vi "MainNR.vi"(10 "JQMHStartup":refnum<class "RQMHStartup.lvclass">, 11 "NewTemplate in":refnum<class "UIManager.lvclass">) -> ()   [LabVIEW 2024, in "UIManager.lvclass"]
uses:
  UIManager.lvclass
  C:/Github/JQMH/JQMHCore/Module/RQMHModule.lvclass
  JQMHCore/JQMHStartup/RQMHStartup.lvclass
  Shell/Shell.lvclass
  Layout/Layout.lvclass
  JQMHCore/Module/RQMHModule.lvclass
  Message Queue_class/RQMHMessageQueue.lvclass/RQMHMessageQueue.ctl
  JQMHCore/Module/InitialiseReplyArgs.ctl
  <vilib>/Utility/miscctls.llb/LVPointTypeDef.ctl
  JQMHCore/Module/RQMHModule.lvclass/RQMHModule.ctl
  Do Something ReplyArgs.ctl
  Do Something Args.ctl
  Prepare Args.ctl
  Prepare ReplyArgs.ctl
  Show ReplyArgs.ctl
  Show Args.ctl
  Add Eng Panel Args.ctl
  Add Eng Panel ReplyArgs.ctl
  Message Queue_class/Delacor_lib_QMH_Enqueue Message (Single).vi
  JQMHCore/Module/Read ModuleName.vi
  JQMHCore/Module/Read External Start.vi
  TitleBar/TitleBar.lvclass
  Header/Header.lvclass
  JQMHCore/Module/Show In Subpanel.vi
  JQMHCore/Module/Show Front Panel.vi
  Message Queue_class/RQMHMessageQueue.lvclass
  JQMHCore/Shared/RQMHShared.lvlib
  C:/Github/JQMH/ModuleTemplates/TitleBar/TitleBar.lvclass
  C:/Github/JQMH/ModuleTemplates/Header/Header.lvclass
  C:/Github/JQMH/ModuleTemplates/Shell/Shell.lvclass
  C:/Github/JQMH/ModuleTemplates/Layout/Layout.lvclass
panel:
  out "error out":errorcluster
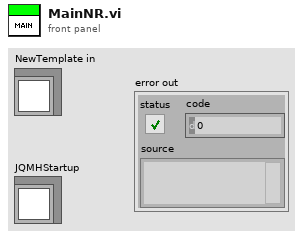
[diagram p1: front panel]
types:
  T1 = typedef "RQMHModule.lvclass/StandardBroadcasts.ctl" = cluster{"Died":refnum<user-event>, "Started":refnum<user-event>}
  T2 = typedef "Header.lvclass/Broadcast Events--cluster.ctl" = cluster{"Stopped":refnum<user-event>, "Menu Item Selected":refnum<user-event>}
  T3 = typedef "TitleBar.lvclass/Broadcast Events--cluster.ctl" = cluster{"Stopped":refnum<user-event>, "Maximise":refnum<user-event>, "Minimise":refnum<user-event>, "ClosePress":refnum<user-event>}
  T4 = typedef "UIManager.lvclass/Request Events--cluster.ctl" = cluster{"Do Something":refnum<user-event>, "Prepare":refnum<user-event>, "Show":refnum<user-event>, "AddEngPanel":refnum<user-event>, "Add Eng Panel":refnum<user-event>}
  T5 = cluster{"Stop Module":refnum<user-event>, "Requests":T4}
  T6 = cluster{"Shell":refnum<class "Shell.lvclass">, "Layout":refnum<class "Layout.lvclass">, "TitleBar":refnum<class "TitleBar.lvclass">, "Header":refnum<class "Header.lvclass">, "EngPanels":map{string, refnum<class "RQMHModule.lvclass">}}
  T7 = typedef "LVPointTypeDef.ctl" = cluster{"Horizontal":i16, "Vertical":i16}
  T8 = enum32{"Invalid", "Standard", "Closed", "Hidden", "Minimized", "Maximized"}
  T9 = typedef "RQMHModule.lvclass/InitialiseReplyArgs.ctl" = cluster{"Did Init?":bool}
  T10 = typedef "UIManager.lvclass/Do Something Args.ctl" = cluster{"Msg":string}
  T11 = typedef "UIManager.lvclass/Do Something ReplyArgs.ctl" = cluster{"Value":dbl, "Boolean":bool}
  T12 = typedef "UIManager.lvclass/Prepare ReplyArgs.ctl" = cluster{"null":bool}
  T13 = typedef "UIManager.lvclass/Prepare Args.ctl" = cluster{"String":string}
  T14 = typedef "UIManager.lvclass/Show Args.ctl" = cluster{"String":string}
  T15 = typedef "UIManager.lvclass/Show ReplyArgs.ctl" = cluster{"Boolean":bool}
  T16 = typedef "UIManager.lvclass/Add Eng Panel ReplyArgs.ctl" = cluster{"null":bool}
  T17 = typedef "UIManager.lvclass/Add Eng Panel Args.ctl" = cluster{"EngPanel":refnum<class "RQMHModule.lvclass">, "Name":string}
  T18 = typedef "RQMHModule.lvclass/Reply.ctl" = cluster{"Expects Reply":bool, "Reply":refnum<notifier>}
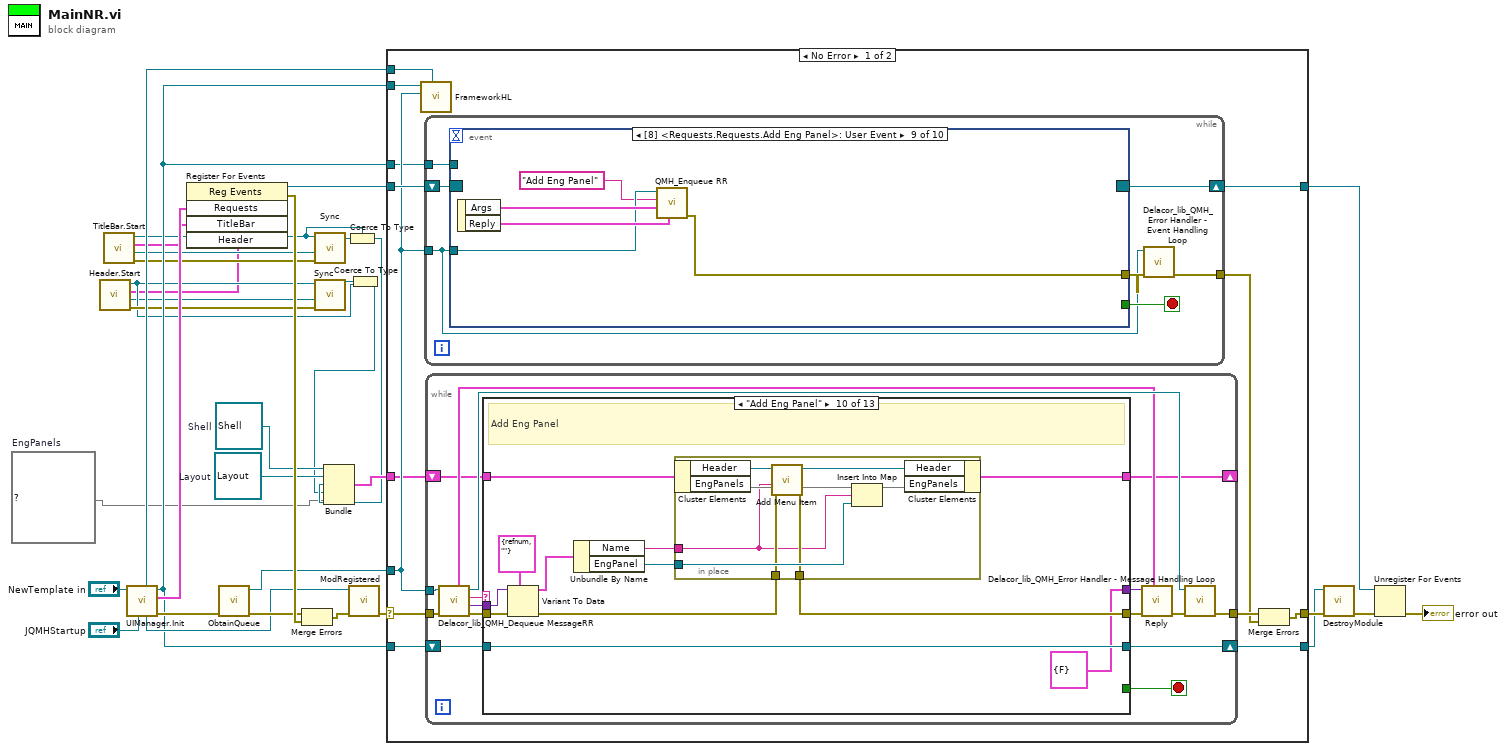
[diagram p0: block diagram]
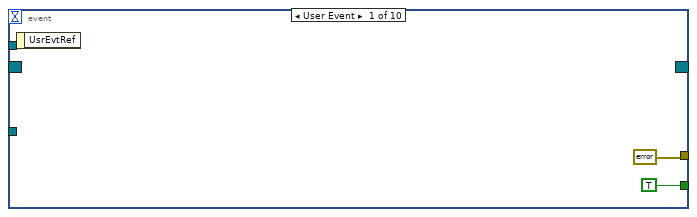
[diagram p2: hidden frame]
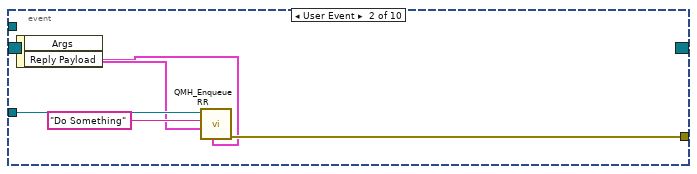
[diagram p3: hidden frame]
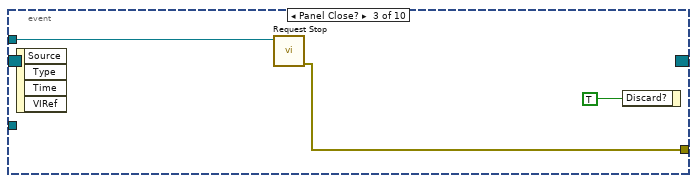
[diagram p4: hidden frame]
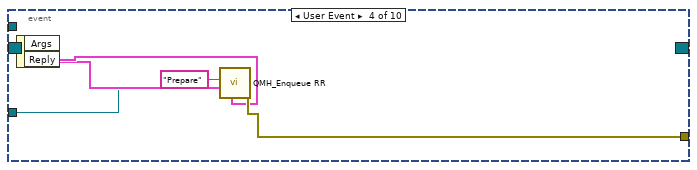
[diagram p5: hidden frame]
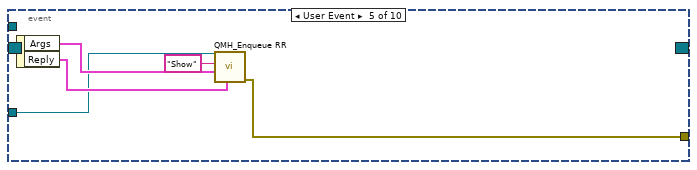
[diagram p6: hidden frame]
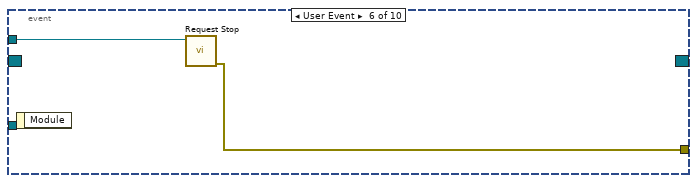
[diagram p7: hidden frame]
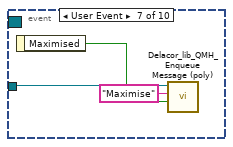
[diagram p8: hidden frame]
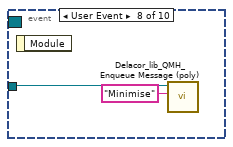
[diagram p9: hidden frame]
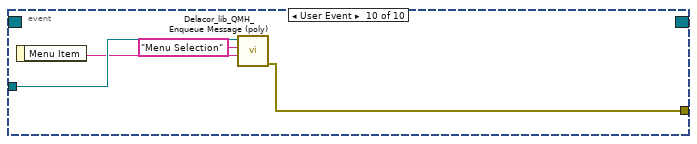
[diagram p10: hidden frame]
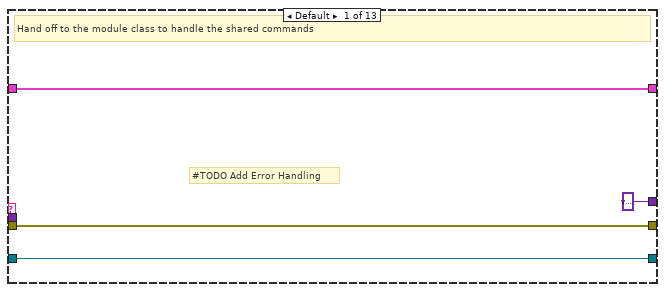
[diagram p11: hidden frame]
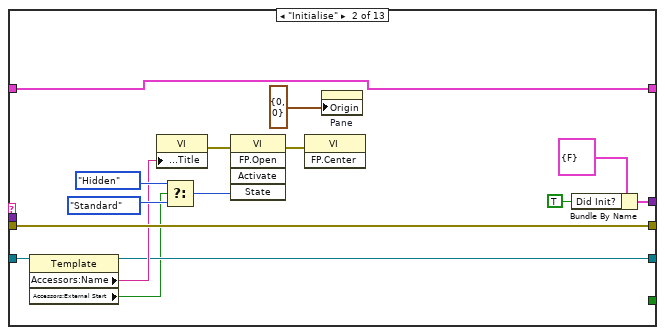
[diagram p12: hidden frame]
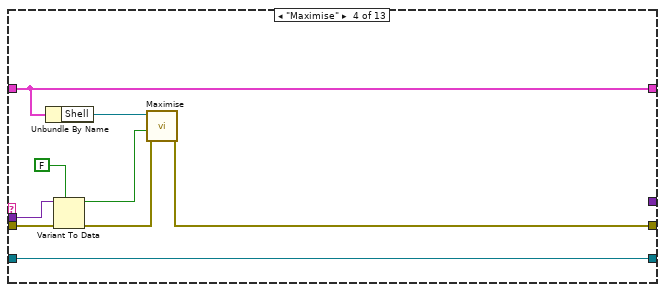
[diagram p14: hidden frame]
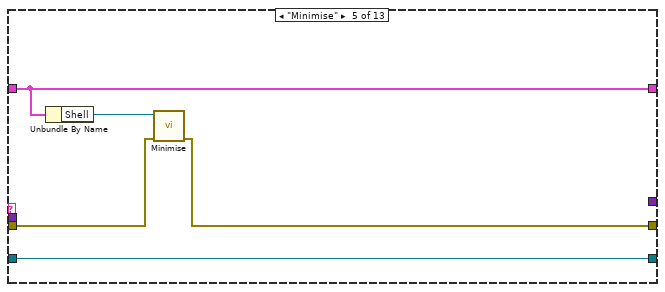
[diagram p15: hidden frame]
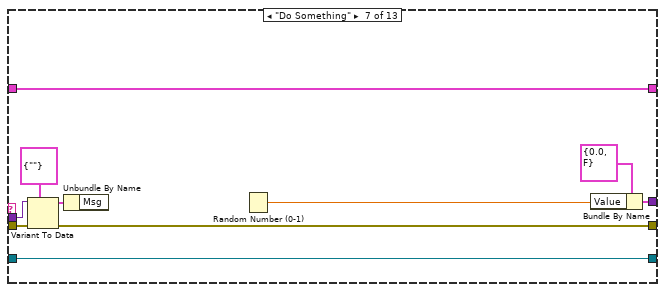
[diagram p17: hidden frame]
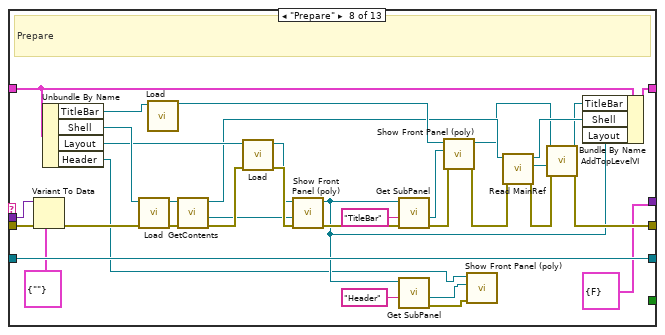
[diagram p18: hidden frame]
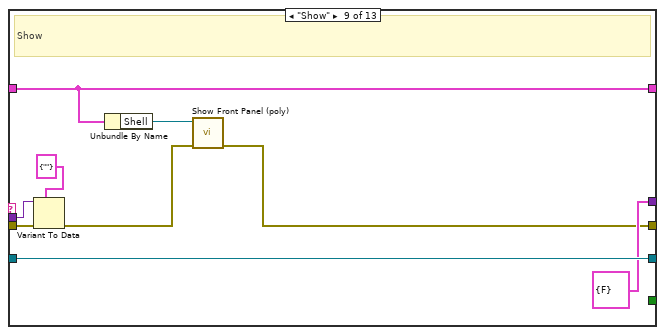
[diagram p19: hidden frame]
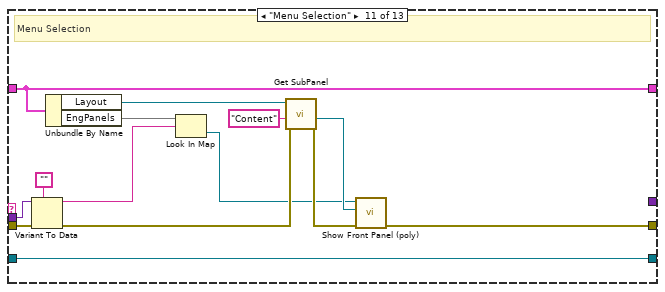
[diagram p20: hidden frame]
diagram:
  w2 = map{string, refnum<class "RQMHModule.lvclass">} {}  # EngPanels
  w14 = refnum<class "Layout.lvclass"> refnum  # Layout
  w16 = refnum<class "Shell.lvclass"> refnum  # Shell
  n1 = call "Header.Start.vi"() -> ("error out"=w5:errorcluster, "StartupHandshake out"=w3:refnum<class "RQMHStartup.lvclass">, 2:"Header"=w1:cluster{"Broadcasts":T1, "Broadcasts":T2}, 3:"Header"=w4:refnum<class "Header.lvclass">)  [unwired: 8 in]
  n2 = call "TitleBar.Start.vi"() -> ("error out"=w11:errorcluster, "StartupHandshake out"=w12:refnum<class "RQMHStartup.lvclass">, 2:"TitleBar"=w13:cluster{"Broadcasts":T1, "Broadcasts":T3}, 3:"TitleBar"=w8:refnum<class "TitleBar.lvclass">)  [unwired: 8 in]
  n3 = call "UIManager.Init.vi"("JQMHStartup in"="JQMHStartup", "NewTemplate in"="NewTemplate in") -> ("error out"=w27:errorcluster, "Requests"=w18:T5, "NewTemplate out"=w17:refnum<class "UIManager.lvclass">, "JQMHStartup out"=w25:refnum<class "RQMHStartup.lvclass">, "StandardRequests"=w21:refnum<event-registration>)  [unwired: 4 in, 1 out]
  n4 = register-events(w18, w13, w1) -> (reference out=w20:refnum<event-registration>, error out=w34:errorcluster)  [unwired: 2 in]
  n5 = call "ObtainQueue.vi"("error in"=w27) -> ("error out"=w26:errorcluster, "Message Queue"=w22:refnum<class "RQMHMessageQueue.lvclass">)  [unwired: 9 in]
  n6 = Merge Errors(w26, w34) -> (w23:errorcluster)
  n7 = call "Sync.vi"("error in (no error)"=w11, "StartupHandshake out"=w12, "JQMHCore in"=w8) -> ("JQMHCore out"=w9:refnum<class "TitleBar.lvclass">)  [unwired: 7 in, 1 out]
  n8 = call "Sync.vi"("error in (no error)"=w5, "StartupHandshake out"=w3, "JQMHCore in"=w4) -> ("JQMHCore out"=w6:refnum<class "Header.lvclass">)  [unwired: 7 in, 1 out]
  n9 = Coerce To Type(0:w9, 1:w8) -> (2:w10:refnum<class "TitleBar.lvclass">)
  n10 = call "ModRegistered.vi"("error in (no error)"=w23, "JQMHStartup in"=w25) -> ("error out"=w24:errorcluster)  [unwired: 9 in]
  n11 = Coerce To Type(0:w6, 1:w4) -> (2:w7:refnum<class "Header.lvclass">)
  n12 = Bundle("Shell"=w16, "Layout"=w14, "TitleBar"=w10, "Header"=w7, "EngPanels"=w2) -> (w15:T6)  [unwired: 1 in]
  n13 = case "RQMH_MAIN" shown="No Error" w24 {
    selector: w24 -> [w44 w257]
    tunnel: w17 -> [w47 w256]
    tunnel: [w46 w259] -> w33
    tunnel: w20 -> [w45 w259]
    tunnel: w22 -> [w38 w258]
    tunnel: [w43 w256] -> w19
    tunnel: [w40 w255] -> w30
    tunnel: w17 -> [w39 _]
    tunnel: w21 -> [w37 w254]
    tunnel: w17 -> [w36 _]
    tunnel: w15 -> [w35 _]
    frame No Error {
      n14 = call-dynamic "FrameworkHL.vi"("StandardRequests"=w37, "Message Queue"=w38, "JQMHModule in"=w39) -> ()  [unwired: 9 in]
      n15 = while {
        shift-right: [w54] -> w46
        shift-left: w45 -> [w49]
        tunnel: w38 -> [w50]
        tunnel: [w51] -> w41
        tunnel: w36 -> [w48]
        stop <- w53 stop-if-true
        n16 = event "RQMH_EVENT_MAIN" shown="[8] <Requests.Requests.Add Eng Panel>: User Event" {
          selector: w49 -> [_ _ _ _ _ _ _ _ _ _]
          dyn-events: [_ _ _ _ _ _ _ _ _ _] -> w54
          timeout: _ -> [_ _ _ _ _ _ _ _ _ _]
          tunnel: [TRUE _ _ _ _ _ _ _ _ _] -> w53
          tunnel: w50 -> [_ w61 _ w66 w71 _ w79 w81 w83 w90]
          tunnel: [errorcluster {"status"=FALSE, "code"=0, "source"=""} ("error out") w58 w62 w69 w74 w75 _ _ w86 w87] -> w52
          tunnel: w48 -> [_ _ w63 _ _ w76 _ _ _ _]
          event User Event {
            n17 = event-data() -> ()  [unwired: 1 in, 1 out]
          }
          event User Event {
            n18 = event-data() -> ("Args"=w59:T10, "Reply Payload"=w57:T18)  [unwired: 1 in]
            n19 = call "QMH_Enqueue RR.vi"("Reply"=w57, "Message Data"=w59, "Message"="Do Something", "Message Queue in"=w61) -> ("error out"=w58:errorcluster)  [unwired: 6 in, 1 out]
          }
          event Panel Close? {
            n20 = event-data() -> ()  [unwired: 1 in, 4 out]
            n21 = call "Request Stop.vi"("module in"=w63) -> ("error out"=w62:errorcluster)  [unwired: 9 in, 1 out]
            n22 = event-data("Discard?"=TRUE) -> ()  [unwired: 1 in, 1 out]
          }
          event User Event {
            n23 = event-data() -> ("Args"=w67:T13, "Reply"=w68:T18)  [unwired: 1 in]
            n24 = call "QMH_Enqueue RR.vi"("Reply"=w68, "Message Data"=w67, "Message"="Prepare", "Message Queue in"=w66) -> ("error out"=w69:errorcluster)  [unwired: 6 in, 1 out]
          }
          event User Event {
            n25 = event-data() -> ("Args"=w72:T14, "Reply"=w73:T18)  [unwired: 1 in]
            n26 = call "QMH_Enqueue RR.vi"("Reply"=w73, "Message Data"=w72, "Message"="Show", "Message Queue in"=w71) -> ("error out"=w74:errorcluster)  [unwired: 6 in, 1 out]
          }
          event User Event {
            n27 = event-data() -> ()  [unwired: 1 in, 1 out]
            n28 = call "Request Stop.vi"("module in"=w76) -> ("error out"=w75:errorcluster)  [unwired: 9 in, 1 out]
          }
          event User Event {
            n29 = event-data() -> ("Maximised"=w77:bool)  [unwired: 1 in]
            n30 = call-poly "Delacor_lib_QMH_Enqueue Message (poly).vi"("Message Data"=w77, "Message"="Maximise", "Message Queue in"=w79) -> ()  [unwired: 7 in, 2 out]
          }
          event User Event {
            n31 = event-data() -> ()  [unwired: 1 in, 1 out]
            n32 = call-poly "Delacor_lib_QMH_Enqueue Message (poly).vi"("Message"="Minimise", "Message Queue in"=w81) -> ()  [unwired: 8 in, 2 out]
          }
          event User Event {
            n33 = event-data() -> ("Args"=w84:T17, "Reply"=w85:T18)  [unwired: 1 in]
            n34 = call "QMH_Enqueue RR.vi"("Reply"=w85, "Message Data"=w84, "Message"="Add Eng Panel", "Message Queue in"=w83) -> ("error out"=w86:errorcluster)  [unwired: 6 in, 1 out]
          }
          event User Event {
            n35 = event-data() -> ("Menu Item"=w89:string)  [unwired: 1 in]
            n36 = call-poly "Delacor_lib_QMH_Enqueue Message (poly).vi"("Message Data"=w89, "Message"="Menu Selection", "Message Queue in"=w90) -> ("error out"=w87:errorcluster)  [unwired: 7 in, 1 out]
          }
        }
        n37 = call-dynamic "Delacor_lib_QMH_Error Handler - Event Handling Loop.vi"("error in"=w52, "Message Queue in"=w50) -> ("dup error in"=w51:errorcluster)  [unwired: 8 in, 1 out]
      }
      n38 = while {
        tunnel: w38 -> [w101]
        tunnel: w44 -> [w100]
        shift-right: [w103] -> w43
        shift-left: w47 -> [w104]
        tunnel: [w102] -> w42
        shift-right: [w91] -> _
        shift-left: w35 -> [w92]
        stop <- w106 stop-if-true
        n39 = call-dynamic "Delacor_lib_QMH_Dequeue MessageRR.vi"("error in"=w100, "Message Queue in"=w101) -> ("error out"=w99:errorcluster, "Message Data"=w97:variant, "Message"=w98:string, "Message Queue out"=w105:refnum<class "RQMHMessageQueue.lvclass">, "Reply"=w93:T18)  [unwired: 5 in]
        n40 = case "RQMH_MESSAGE_CASES" shown="\"Add Eng Panel\"" w98 {
          tunnel: [_ _ _ _ _ _ _ _ _ _ _ _ TRUE] -> w106
          tunnel: w104 -> [w109 w113 w127 w136 w142 w144 w155 w189 w198 w210 w232 w238 w252]
          tunnel: w97 -> [_ _ _ w134 _ _ w151 w188 w197 w209 w231 w236 _]
          tunnel: w99 -> [w110 w125 w128 w137 w138 w145 w150 w190 w199 w211 w233 w240 w251]
          tunnel: [w110 w125 w128 w130 w139 w145 w149 w164 w191 w201 w221 w239 w251] -> w96
          tunnel: [w109 w114 w127 w136 w142 w144 w155 w189 w198 w210 w232 w237 w252] -> w103
          tunnel: [variant w124 _ _ _ _ w154 T12 {"null"=FALSE} ("Prepare ReplyArgs") T15 {"Boolean"=FALSE} ("RQMH_MHL_REPLY_PL") T16 {"null"=FALSE} _ w235 _] -> w94
          tunnel: w92 -> [w107 w111 w126 w135 w141 w143 w146 w184 w194 w208 w229 w234 w250]
          tunnel: [w107 w111 w126 w135 w141 w143 w146 w185 w194 w205 w229 w234 w250] -> w91
          frame Default {
            # "#TODO Add Error Handling"
            # "Hand off to the module class to handle the shared commands"
          }
          frame "Initialise" {
            n41 = property class="Template"(reference=w113) -> (reference out=w114:refnum<class "UIManager.lvclass">, "Accessors:Name"=w115:string, "Accessors:External Start"=w112:bool)  [unwired: 1 in, 1 out]
            n42 = property on="Property Node" class="VI"("Front Panel.Title"=w115) -> (error out=w122:errorcluster)  [unwired: 2 in, 1 out]
            n43 = Select(t=T8."Hidden" ("State"), s=w112, f=T8."Standard" ("State")) -> (s? t:f=w118:T8)
            n44 = invoke on="Invoke Node" class="VI" method="FP.Open"(error in=w122, "State"=w118) -> (error out=w121:errorcluster)  [unwired: 3 in, 4 out]
            n45 = invoke on="Invoke Node" class="VI" method="FP.Center"(error in=w121) -> ()  [unwired: 2 in, 3 out]
            n46 = property on="Pane" class="Pane"("Origin"=T7 {"Horizontal"=0, "Vertical"=0}) -> ()  [unwired: 2 in, 2 out]
            n47 = Bundle By Name(cluster=T9 {"Did Init?"=FALSE} ("Args"), "Did Init?"=TRUE) -> (w124:T9)
          }
          frame "---Internal---" {
          }
          frame "Maximise" {
            n48 = Unbundle By Name(w135) -> ("Shell"=w132:refnum<class "Shell.lvclass">)
            n49 = Variant To Data(error in=w137, type=FALSE, Variant=w134) -> (data=w129:bool, error out=w131:errorcluster)
            n50 = call "Maximise.vi"("error in (no error)"=w131, "Maximise"=w129, "module in"=w132) -> ("error out"=w130:errorcluster)  [unwired: 6 in, 2 out]
          }
          frame "Minimise" {
            n51 = Unbundle By Name(w141) -> ("Shell"=w140:refnum<class "Shell.lvclass">)
            n52 = call "Minimise.vi"("error in (no error)"=w138, "module in"=w140) -> ("error out"=w139:errorcluster)  [unwired: 7 in, 2 out]
          }
          frame "---Module Specific---" {
          }
          frame "Do Something" {
            n53 = Variant To Data(error in=w150, type=T10 {"Msg"=""} ("Do Something Args"), Variant=w151) -> (data=w147:T10, error out=w149:errorcluster)
            n54 = Unbundle By Name(w147) -> ()  [unwired: 1 out]
            n55 = Random Number (0-1)() -> (number: 0 to 1=w152:dbl)
            n56 = Bundle By Name(cluster=T11 {"Value"=0.0, "Boolean"=FALSE}, "Value"=w152) -> (w154:T11)
          }
          frame "Prepare" {
            # "Prepare"
            n57 = Variant To Data(error in=w190, type=T13 {"String"=""} ("RQMH_MHL_MSG_PL"), Variant=w188) -> (error out=w186:errorcluster)  [unwired: 1 out]
            n58 = Unbundle By Name(w184) -> ("TitleBar"=w175:refnum<class "TitleBar.lvclass">, "Shell"=w183:refnum<class "Shell.lvclass">, "Layout"=w182:refnum<class "Layout.lvclass">, "Header"=w158:refnum<class "Header.lvclass">)
            n59 = call "Load.vi"("error in (no error)"=w186, "RQMHModule in"=w183) -> ("error out"=w180:errorcluster, "RQMHModule out"=w181:refnum<class "Shell.lvclass">)  [unwired: 8 in]
            n60 = call "Load.vi"("RQMHModule in"=w175) -> ("RQMHModule out"=w172:refnum<class "TitleBar.lvclass">)  [unwired: 9 in, 1 out]
            n61 = call "GetContents.vi"("error in (no error)"=w180, "module in"=w181) -> ("error out"=w179:errorcluster, "Sub Panel"=w177:refnum<vi>, "module out"=w168:refnum<class "Shell.lvclass">)  [unwired: 6 in, 1 out]
            n62 = call "Load.vi"("error in (no error)"=w179, "RQMHModule in"=w182) -> ("error out"=w178:errorcluster, "RQMHModule out"=w176:refnum<class "Layout.lvclass">)  [unwired: 8 in]
            n63 = call-poly "Show Front Panel (poly).vi"("error in (no error)"=w178, "Sub Panel"=w177, "JQMHCore in"=w176) -> ("error out"=w174:errorcluster, "JQMHCore out"=w159:refnum<class "Layout.lvclass">)  [unwired: 7 in]
            n64 = call "Get SubPanel.vi"("error in (no error)"=w174, "Panel Name"="TitleBar", "module in"=w159) -> ("error out"=w170:errorcluster, "Sub Panel"=w171:refnum<vi>)  [unwired: 5 in, 2 out]
            n65 = call "Get SubPanel.vi"("Panel Name"="Header", "module in"=w159) -> ("error out"=w156:errorcluster, "Sub Panel"=w157:refnum<vi>)  [unwired: 6 in, 2 out]
            n66 = call-poly "Show Front Panel (poly).vi"("error in (no error)"=w170, "Sub Panel"=w171, "JQMHCore in"=w172) -> ("error out"=w163:errorcluster, "JQMHCore out"=w166:refnum<class "TitleBar.lvclass">)  [unwired: 7 in]
            n67 = call-poly "Show Front Panel (poly).vi"("error in (no error)"=w156, "Sub Panel"=w157, "JQMHCore in"=w158) -> ()  [unwired: 7 in, 2 out]
            n68 = call "Read MainRef.vi"("error in (no error)"=w163, "RQMHModule in"=w168) -> ("error out"=w162:errorcluster, "MainRef"=w169:refnum<vi>, "RQMHModule out"=w167:refnum<class "Shell.lvclass">)  [unwired: 7 in]
            n69 = call "AddTopLevelVI.vi"("error in (no error)"=w162, "MainRef"=w169, "module in"=w166) -> ("error out"=w164:errorcluster, "module out"=w165:refnum<class "TitleBar.lvclass">)  [unwired: 6 in, 1 out]
            n70 = Bundle By Name(cluster=w184, "TitleBar"=w165, "Shell"=w167, "Layout"=w159) -> (w185:T6)
          }
          frame "Show" {
            # "Show"
            n71 = Variant To Data(error in=w199, type=T14 {"String"=""} ("RQMH_MHL_MSG_PL"), Variant=w197) -> (error out=w192:errorcluster)  [unwired: 1 out]
            n72 = Unbundle By Name(w194) -> ("Shell"=w193:refnum<class "Shell.lvclass">)
            n73 = call-poly "Show Front Panel (poly).vi"("error in (no error)"=w192, "JQMHCore in"=w193) -> ("error out"=w191:errorcluster)  [unwired: 8 in, 1 out]
          }
          frame "Add Eng Panel" {
            # "Add Eng Panel"
            n74 = Variant To Data(error in=w211, type=T17 {"EngPanel"=refnum, "Name"=""} ("RQMH_MHL_MSG_PL"), Variant=w209) -> (data=w206:T17, error out=w202:errorcluster)
            n75 = Unbundle By Name(w206) -> ("Name"=w204:string, "EngPanel"=w203:refnum<class "RQMHModule.lvclass">)
            n76 = in-place {
              in-place-border: w204 -> [w212]
              in-place-border: w203 -> [w217]
              in-place-border: w202 -> [w214]
              in-place-border: [w213] -> w201
              n77 = in-place-cluster #1(w208) -> ("Header"=w216:refnum<class "Header.lvclass">, "EngPanels"=w219:map{string, refnum<class "RQMHModule.lvclass">})
              n78 = call "Add Menu Item.vi"("error in (no error)"=w214, "Item"=w212, "module in"=w216) -> ("error out"=w213:errorcluster, "module out"=w215:refnum<class "Header.lvclass">)  [unwired: 7 in]
              n79 = Insert Into Map(map in=w219, key=w212, value=w217) -> (map out=w218:map{string, refnum<class "RQMHModule.lvclass">})  [unwired: 2 out]
              n80 = in-place-cluster #1("Header"=w215, "EngPanels"=w218) -> (w205:T6)
            }
          }
          frame "Menu Selection" {
            # "Menu Selection"
            n81 = Variant To Data(error in=w233, type="", Variant=w231) -> (data=w227:string, error out=w223:errorcluster)
            n82 = Unbundle By Name(w229) -> ("Layout"=w224:refnum<class "Layout.lvclass">, "EngPanels"=w228:map{string, refnum<class "RQMHModule.lvclass">})
            n83 = Look In Map(map=w228, key=w227) -> (value=w220:refnum<class "RQMHModule.lvclass">)  [unwired: 1 in, 1 out]
            n84 = call "Get SubPanel.vi"("error in (no error)"=w223, "Panel Name"="Content", "module in"=w224) -> ("error out"=w222:errorcluster, "Sub Panel"=w226:refnum<vi>)  [unwired: 5 in, 2 out]
            n85 = call-poly "Show Front Panel (poly).vi"("error in (no error)"=w222, "Sub Panel"=w226, "JQMHCore in"=w220) -> ("error out"=w221:errorcluster)  [unwired: 7 in, 1 out]
          }
          frame "---Copy This Frame---" {
            # "This is the frame that is copied when scripting\nDO NOT CHANGE NAME OF FRAME"
            n86 = disable-structure shown="Disabled" {
              disable-tunnel: w240 -> [w244 w249]
              disable-tunnel: [w245 w249] -> w239
              disable-tunnel: w238 -> [w247 w248]
              disable-tunnel: [w247 w248] -> w237
              disable-tunnel: w236 -> [w246 _]
              disable-tunnel: [w242 _] -> w235
              frame Disabled {
                # "Anything in this diagram will be used when adding a new request"
                n87 = Variant To Data(error in=w244, type=cluster{string} {""} ("RQMH_MHL_MSG_PL"), Variant=w246) -> (error out=w245:errorcluster)  [unwired: 1 out]
                n88 = Bundle By Name(cluster=cluster{string} {""} ("RQMH_MHL_REPLY_PL")) -> (w242:cluster{string})  [unwired: 1 in]
              }
              frame Enabled {
              }
            }
          }
          frame "Exit" {
            # "Clean up and send message to EHL"
          }
        }
        n89 = call "Reply.vi"("Reply"=w93, "error in (no error)"=w96, "ReplyPayload"=w94) -> ("error out"=w95:errorcluster)  [unwired: 8 in]
        n90 = call-dynamic "Delacor_lib_QMH_Error Handler - Message Handling Loop.vi"("error in"=w95, "Message Queue in"=w105) -> ("dup error in"=w102:errorcluster)  [unwired: 8 in, 1 out]
      }
      n91 = Merge Errors(w42, w41) -> (w40:errorcluster)
    }
    frame Error {
      n92 = call-dynamic "Delacor_lib_QMH_Release Message Queue.vi"("error in"=w257, "Message Queue"=w258) -> ("error out"=w255:errorcluster)  [unwired: 9 in]
      n93 = Unregister For Events(event registration refnum=w254) -> ()  [unwired: 1 in, 1 out]
    }
  }
  n94 = call "DestroyModule.vi"("error in (no error)"=w30, "JQMHModule in"=w19) -> ("error out"=w32:errorcluster)  [unwired: 9 in]
  n95 = Unregister For Events(event registration refnum=w33, error in=w32) -> (error out=→"error out":errorcluster)
